vi "Override To Normal.vi"(11 "Base Actor in":refnum<class "Base Actor.lvclass">) -> (3 "Base Actor out":refnum<class "Base Actor.lvclass">)   [LabVIEW 2021, in "jettl.lvlib" / "Actor.lvlib" / "Base Actor.lvclass"]
uses:
  Base Actor.lvclass
  Base Actor.lvclass/Base Actor.ctl
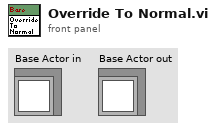
[diagram p1: front panel]
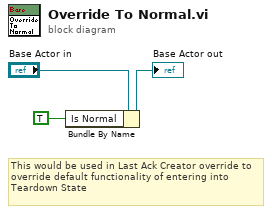
[diagram p0: block diagram]
diagram:
  # "This would be used in Last Ack Creator override to override default functionality of entering into Teardown State"
  n1 = Bundle By Name(cluster="Base Actor in", "Is Normal"=TRUE) -> (→"Base Actor out":refnum<class "Base Actor.lvclass">)
